vi "Joystick to Swerve.vi"(9 "Joystick R":dbl, 10 "Joystick Y":dbl, 11 "Joystick X":dbl) -> (0 "RearRight Angle (deg)":dbl, 1 "RearRight Power":dbl, 2 "FrontRight Angle (deg)":dbl, 3 "FrontRight Power":dbl, 4 "RearLeft Power":dbl, 5 "FrontLeft Power":dbl, 6 "RearLeft Angle (deg)":dbl, 7 "FrontLeft Angle (deg)":dbl)   [LabVIEW 2016]
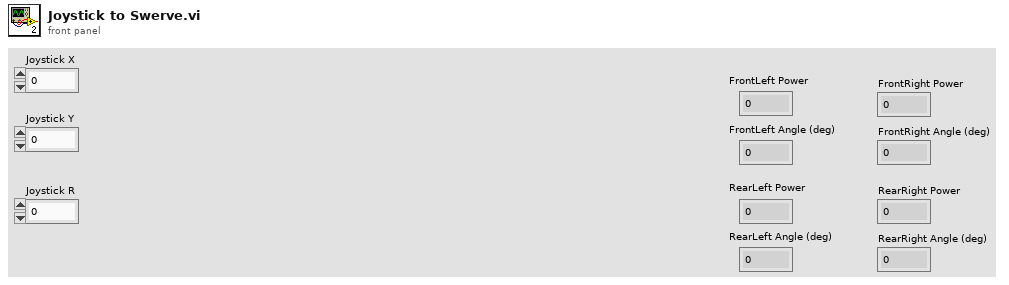
[diagram p1: front panel]
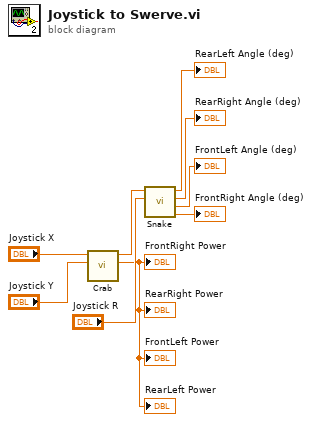
[diagram p0: block diagram]
diagram:
  n1 = call "Crab.vi"("J1 Y"="Joystick Y", "J1 X"="Joystick X") -> ("Magnitude"=→"FrontRight Power" →"FrontLeft Power" →"RearLeft Power" →"RearRight Power":dbl, "Joystick Degree"=w7:dbl)  [unwired: 8 out]
  n2 = call "Snake.vi"("Snake"="Joystick R", "Crab Degree"=w7) -> ("FR"=→"FrontRight Angle (deg)":dbl, "FL"=→"FrontLeft Angle (deg)":dbl, "RR"=→"RearRight Angle (deg)":dbl, "RL"=→"RearLeft Angle (deg)":dbl)  [unwired: 6 out]
